vi "UIRef.vi"(8 "error in":errorcluster, 11 "group in":refnum<class "Group.lvclass">) -> (0 "error out":errorcluster, 2 "VI refnum":refnum<vi>, 3 "group out":refnum<class "Group.lvclass">)   [LabVIEW 2013, in "Group.lvclass"]
uses:
  Group.lvclass
  GroupUI.vi
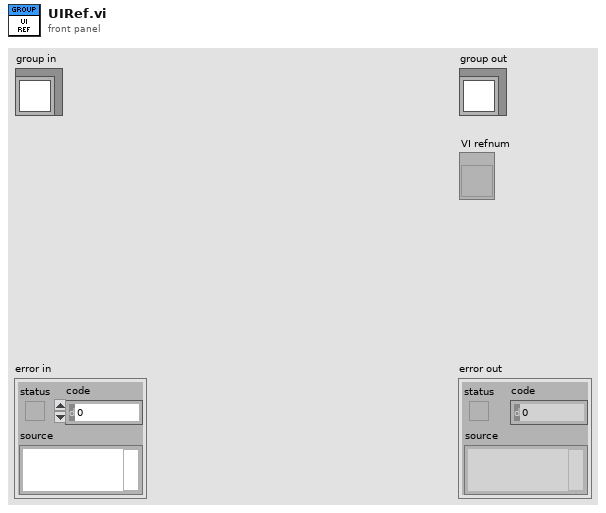
[diagram p1: front panel]
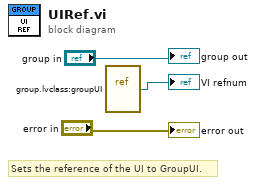
[diagram p0: block diagram]
diagram:
  # "Sets the reference of the UI to GroupUI."
  n1 = vi-ref "group.lvclass:groupUI.vi"() -> (→"VI refnum":refnum<vi>)
  "error out" <- "error in"
  "group out" <- "group in"
